vi "Unpack for gRPC.vi"(8 "error in":errorcluster, 9 "configuration / results":enum16{"Configuration", "Results"}(ring), 10 "any":T1, 11 "measurement customizations in":refnum<class "Measurement Plugin.lvclass">) -> (0 "error out":errorcluster, 2 "data value":variant, 3 "measurement customizations out":refnum<class "Measurement Plugin.lvclass">)   [LabVIEW 2021, in "PSRR_PMIC.lvlib" / "Measurement Plugin.lvclass"]
uses:
  Measurement Plugin.lvclass
  Measurement Plugin.lvclass/Measurement Plugin.ctl
  Measurement Configuration.ctl
  PSRR_PMIC.lvlib
  Measurement Results.ctl
  3ecd018e-d556-4cbc-bc60-c4ba57204520.vi
  a521b266-ce99-437c-923d-067dcf1e07fd.vi
  <vilib>/Plug-In SDKs/Measurements/Measurement Plugin Service/Measurement Plugin Service.lvclass
  C:/Program Files/National Instruments/LabVIEW 2021/vi.lib/Plug-In SDKs/Measurements/Measurement Plugin Service/Measurement Plugin Service.lvclass
  C:/LR/pmic-labview/source/measurements/psrr/PSRR_PMIC/Advanced/Measurement Plugin.lvclass
  <vilib>/gRPC/LabVIEW gRPC Library/Shared/Any.ctl
  <vilib>/gRPC/LabVIEW gRPC Library/grpc-lvsupport-release.lvlib
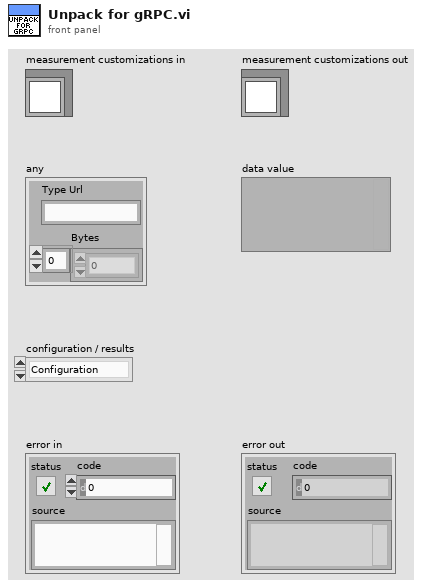
[diagram p1: front panel]
types:
  T1 = typedef "grpc-lvsupport-release.lvlib/Any.ctl" = cluster{"Type Url":string, "Bytes":u8[]}
  T2 = typedef "grpc-lvsupport-release.lvlib/grpcId.ctl" = u64
  T3 = typedef "PSRR_PMIC.lvlib/Measurement Configuration.ctl" = cluster{"DUT setup time":dbl, "Source resource name":string, "Source current limit":dbl, "Source voltage level":dbl, "Load resource name":string, "Load voltage limit range":dbl, "Load current level":dbl, "Fgen resource name":string, "Fgen channel name":string, "Fgen amplitude":dbl, "Fgen load impedence":dbl, "Fgen start frequency":dbl, "Fgen stop frequency":dbl, "Fgen frequency sweep points/points per decade":i32, "Fgen sweep type":string, "Fgen standard Waveform":enum16{"Sine", "Square", "Triangle", "Ramp Up", "Ramp Down", "DC", "Noise"}, "Scope resource name":string, "Scope input channel name":string, "Scope output channel name":string, "Scope probe attenuation":dbl, "Scope samples per cycle":u32, "Scope cycles to average":u32}
  T4 = typedef "PSRR_PMIC.lvlib/Measurement Results.ctl" = cluster{"Frequency sweep point":dbl[], "PSRR":dbl[]}
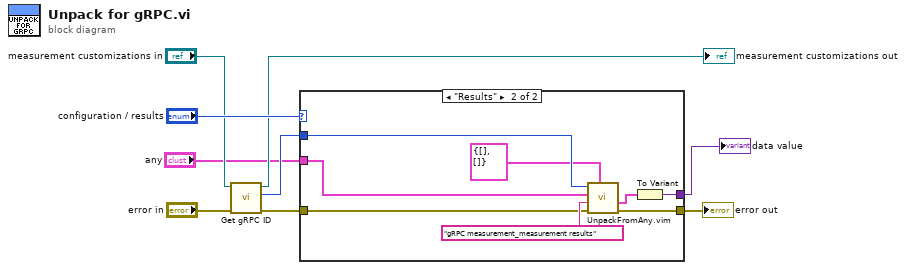
[diagram p0: block diagram]
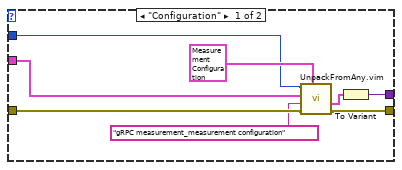
[diagram p2: hidden frame]
diagram:
  n1 = call <vilib>:"Get gRPC ID.vi"("error in"="error in", "measurement plugin service in"="measurement customizations in") -> ("error out"=w6:errorcluster, "gRPC ID"=w3:T2, "measurement plugin service out"=→"measurement customizations out":refnum<class "Measurement Plugin.lvclass">)  [unwired: 7 in]
  n2 = case shown="\"Results\"" "configuration / results" {
    tunnel: w6 -> [w15 w19]
    tunnel: "any" -> [w10 w18]
    tunnel: w3 -> [w12 w22]
    tunnel: [w16 w23] -> w9
    tunnel: [w17 w25] -> w1
    frame "Configuration" {
      n3 = call "UnpackFromAny.vim"("Data Type"=T3 {"DUT setup time"=1.0, "Source resource name"="", "Source current limit"=0.15, "Source voltage level"=10.0, "Load resource name"="", "Load voltage limit range"=6.0, "Load current level"=0.025, "Fgen resource name"="", "Fgen channel name"="", "Fgen amplitude"=1.0, "Fgen load impedence"=10000.0, "Fgen start frequency"=10.0, "Fgen stop frequency"=10000000.0, "Fgen frequency sweep points/points per decade"=10, "Fgen sweep type"="Logarithmic", "Fgen standard Waveform"=enum."Sine", "Scope resource name"="", "Scope input channel name"="", "Scope output channel name"="", "Scope probe attenuation"=1.0, "Scope samples per cycle"=1000, "Scope cycles to average"=4} ("Measurement Configuration"), "error in"=w15, "Message Type"="gRPC measurement_measurement configuration", "Any"=w10, "gRPCid in"=w12) -> ("error out"=w16:errorcluster, "Unpacked Value"=w14:T3)  [unwired: 4 in, 1 out]
      n4 = To Variant(anything=w14) -> (Variant=w17:variant)
    }
    frame "Results" {
      n5 = call "UnpackFromAny.vim"("Data Type"=T4 {"Frequency sweep point"=[], "PSRR"=[]} ("Measurement Results"), "error in"=w19, "Message Type"="gRPC measurement_measurement results", "Any"=w18, "gRPCid in"=w22) -> ("error out"=w23:errorcluster, "Unpacked Value"=w24:T4)  [unwired: 4 in, 1 out]
      n6 = To Variant(anything=w24) -> (Variant=w25:variant)
    }
  }
  "error out" <- w9
  "data value" <- w1
